vi "graph_in.vi"() -> (0 "map":cluster{"x":dbl[], "y":dbl[]}, 1 "y0":dbl[](array[numeric]), 2 "x0":dbl[](array[numeric]))   [LabVIEW 2015]
uses:
  <vilib>/imath/engines/lvmath2/RunTimeEngine/NodeEndStatement/NIMS_NodeEndStatement_Output.vi
  <instcachedir>/0/NIMS_NodeEndStatement_Output_53EC0D466D134D7ABD903AC30B43404B.lvgen/NIMS_NodeEndStatement_Output_53EC0D466D134D7ABD903AC30B43404B_005.vi
  <vilib>/imath/engines/lvmath2/RunTimeEngine/ErrorHandling/NIMS_Finalize Error.vi
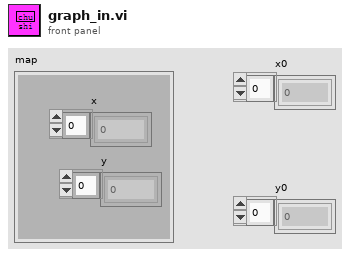
[diagram p1: front panel]
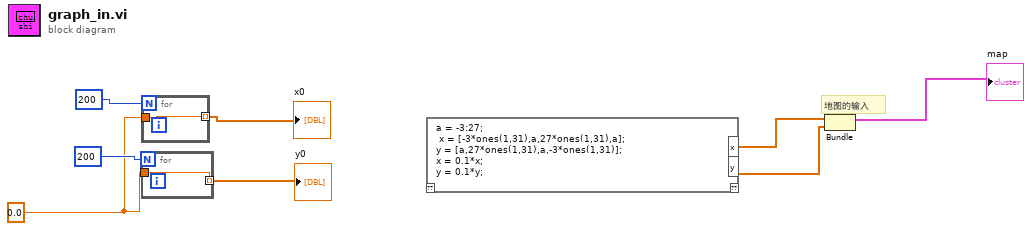
[diagram p0: block diagram]
diagram:
  w6 = 0.0
  # "地图的输入"
  n1 = for {
    N: 200 -> [_]
    tunnel: w6 -> [w9]
    tunnel: [w9] -> w3 mode=indexing
  }
  "y0" <- w3
  n2 = for {
    N: 200 -> [_]
    tunnel: w6 -> [w10]
    tunnel: [w10] -> w4 mode=indexing
  }
  "x0" <- w4
  n3 = mathscript code="a = -3:27;\n x = [-3*ones(1,31),a,27*ones(1,31),a];\ny = [a,27*ones(1,31),a,-3*ones(1,31)];\nx = 0.1*x;\ny = 0.1*y;"() -> ("x"=w2:dbl[], "y"=w1:dbl[])  [unwired: 1 in, 1 out]
  n4 = Bundle("x"=w2, "y"=w1) -> (→"map":cluster{"x":dbl[], "y":dbl[]})  [unwired: 1 in]
